vi "ArrayTo1DString.vi"(8 "ErrorIn(No Error)":errorcluster caption="entrée d'erreur (pas d'erreur)", 9 "Chaîne":string, 10 "DelArrEnd":bool, 11 "tableau":string[][](array[string])) -> (0 "sortie d'erreur":errorcluster, 2 "Size":i32, 3 "Array Out":string[](array[string]))   [LabVIEW 2019]
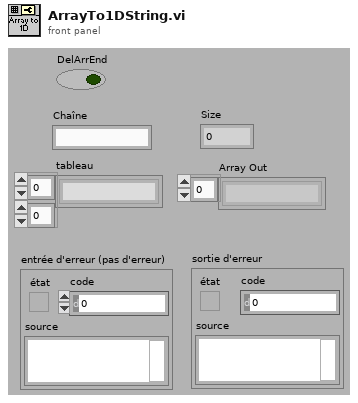
[diagram p1: front panel]
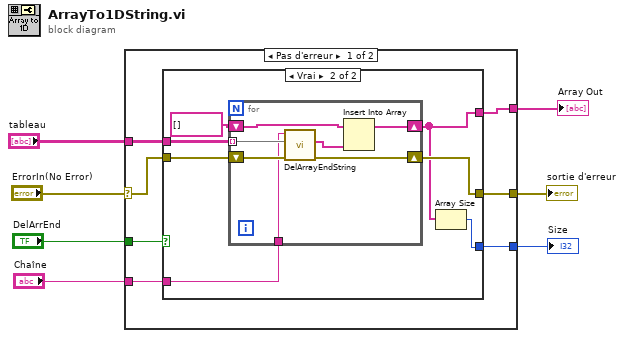
[diagram p0: block diagram]
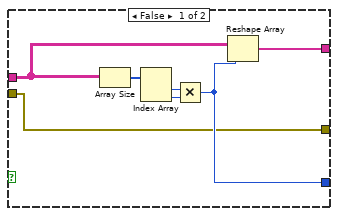
[diagram p2: hidden frame]
diagram:
  n1 = case shown="Pas d'erreur" "ErrorIn(No Error)" {
    selector: "ErrorIn(No Error)" -> [w11 w36]
    tunnel: [w10 w36] -> w6
    tunnel: "tableau" -> [w14 _]
    tunnel: [w13 _] -> w4
    tunnel: [w12 _] -> w3
    tunnel: "DelArrEnd" -> [w9 _]
    tunnel: "Chaîne" -> [w8 _]
    frame No Error {
      n2 = case shown="Vrai" w9 {
        tunnel: w14 -> [w18 w28]
        tunnel: [w17 w24] -> w13
        tunnel: [w16 w23] -> w12
        tunnel: w11 -> [w15 w27]
        tunnel: [w15 w26] -> w10
        tunnel: w8 -> [_ w22]
        frame False {
          n3 = Array Size(array=w18) -> (size(s)=w21:i32[])
          n4 = Index Array(array=w21) -> (element #1=w19:i32, element #2=w20:i32)  [unwired: 2 in]
          n5 = Multiply(x=w19, y=w20) -> (x*y=w17:i32)
          n6 = Reshape Array(w18, w17) -> (w16:string[])
        }
        frame True {
          n7 = for {
            tunnel: w28 -> [w35] mode=indexing
            shift-right: [w33] -> w26
            shift-left: w27 -> [w34]
            shift-right: [w31] -> w23
            shift-left: string[] [] -> [w30]
            tunnel: w22 -> [w29]
            n8 = call <userlib>:"DelArrayEndString.vi"("ErrorIn(No Error)"=w34, "Array In"=w35, "Chaîne"=w29) -> ("sortie d'erreur"=w33:errorcluster, "Array Out"=w32:string[])  [unwired: 7 in]
            n9 = Insert Into Array(array=w30, new element=w32) -> (w31:string[])  [unwired: 1 in]
          }
          n10 = Array Size(array=w23) -> (size(s)=w24:i32)
        }
      }
    }
    frame Error {
    }
  }
  "sortie d'erreur" <- w6
  "Size" <- w4
  "Array Out" <- w3
